vi "CCDAcqSingleSpectrum.vi"(0 "device selection":enum16{"monochromator", "CCD", "SCD"}(ring)=enum."CCD", 1 "ROI":T1, 5 "set-up a connection":bool=TRUE, 9 "tear down connection":bool=TRUE, 11 "error in":errorcluster, 12 "activate logger?":bool, 13 "Handler Name":string="example logger handler") -> (3 "log-file path":path, 6 "ROI cluster":T1, 15 "error out":errorcluster)   [LabVIEW 2023]
uses:
  Classes/CCD/CCDSpectralData.ctl
  Classes/CCD/XAxisConversionTypeEnum.ctl
  Classes/CCD/AcquisitionFormatEnum.ctl
  Classes/CCD/CCD.lvclass
  C:/Projects/Horiba/horiba-labview-sdk/Source/Classes/GenericDevice/GenericDevice.lvclass
  <vilib>/addons/_JKI Toolkits/Caraya/classes/Assert/Assert Not Error.vi
  <vilib>/addons/_JKI Toolkits/Caraya/classes/Test/Test.lvclass
  <vilib>/addons/_JKI Toolkits/Caraya/classes/Assert/Assert.lvclass
panel:
  # "Connector Pane"
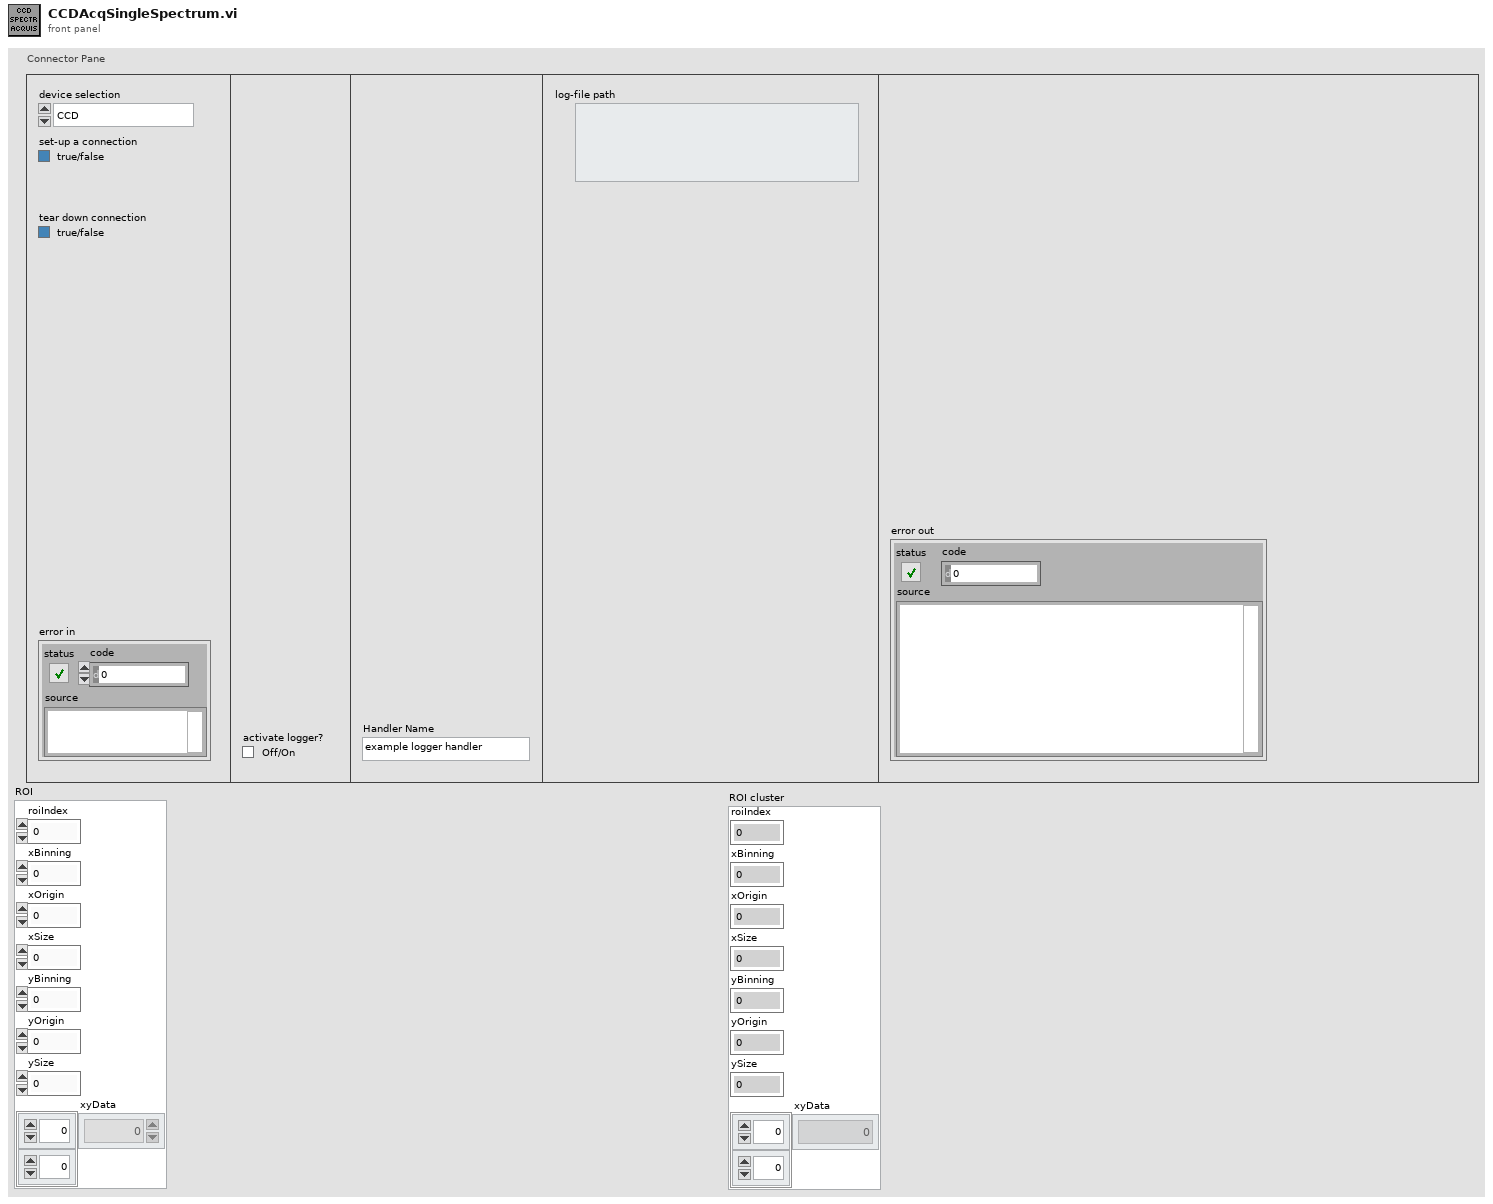
[diagram p1: front panel]
types:
  T1 = typedef "CCD.lvclass/CCDSpectralData.ctl" = cluster{"roiIndex":i32, "xBinning":i32, "xOrigin":i32, "xSize":i32, "yBinning":i32, "yOrigin":i32, "ySize":i32, "xyData":dbl[][]}
  T2 = typedef "CCD.lvclass/AcquisitionFormatEnum.ctl" = enum16{"Spectra", "Image", "Crop", "Fast Kinetics"}
  T3 = typedef "CCD.lvclass/XAxisConversionTypeEnum.ctl" = enum16{"None (default)", "CCD FIT parameters contained in the CCD firmware", "Mono Wavelength parameters contained in the icl_settings.ini file"}
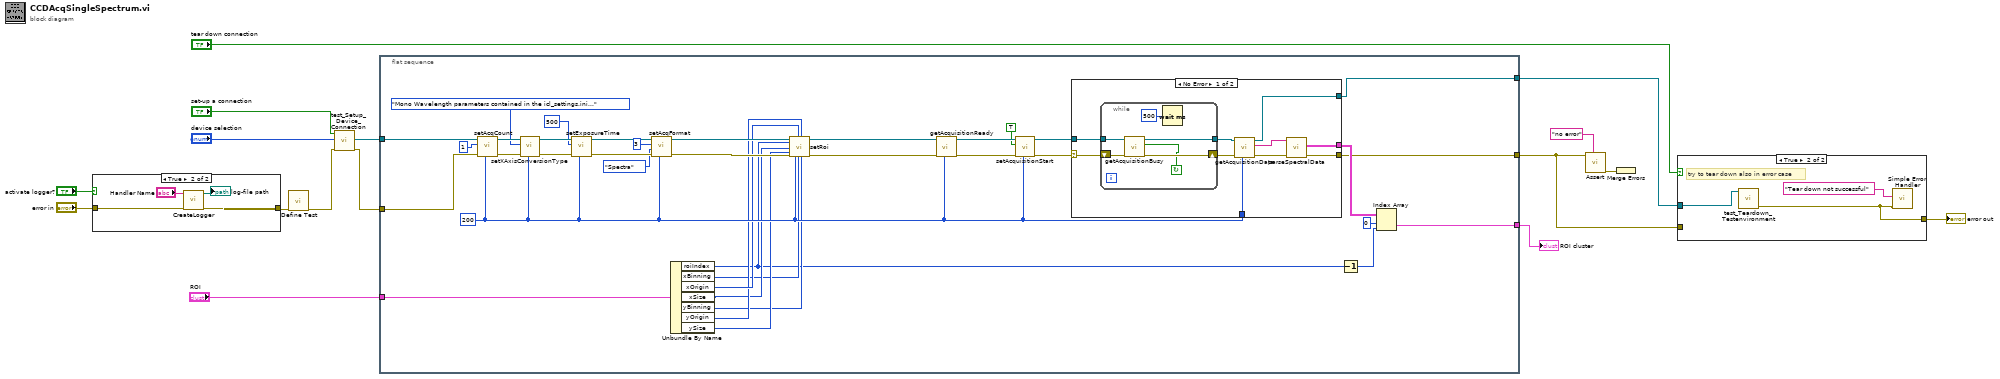
[diagram p0: block diagram]
diagram:
  n1 = case shown="True" "activate logger?" {
    tunnel: [w17 w20] -> w4
    tunnel: "error in" -> [w17 w21]
    frame False {
    }
    frame True {
      n2 = call "CreateLogger.vi"("error in (no error)"=w21, "Handler Name"="Handler Name") -> ("error out"=w20:errorcluster, "log-file path"=→"log-file path":path)  [unwired: 8 in]
    }
  }
  n3 = call <vilib>:"Define Test.vi"("error in (no error)"=w4) -> ("error out"=w9:errorcluster)  [unwired: 9 in, 1 out]
  n4 = call "test_Setup_Device_Connection.vi"("error in (no error)"=w9, "device selection"="device selection", "set-up a connection"="set-up a connection") -> ("error out"=w10:errorcluster, "CCD.lvclass"=w11:refnum<class "CCD.lvclass">)  [unwired: 5 in, 2 out]
  n5 = flat-sequence {
    tunnel: w10 -> [w57]
    tunnel: w11 -> [w58]
    tunnel: [w36] -> w13
    tunnel: [w46] -> w12
    tunnel: [w35] -> w3
    tunnel: "ROI" -> [w32]
    frame #0 {
      w33 = 200 ("Delay between send and receive [ms]")
      n6 = call "setAcqCount.vi"("Delay between send and receive [ms]"=w33, "error in (no error)"=w57, "count"=1, "CCD in"=w58) -> ("error out"=w54:errorcluster, "CCD out"=w55:refnum<class "CCD.lvclass">)  [unwired: 4 in, 2 out]
      n7 = call "setXAxisConversionType.vi"("Delay between send and receive [ms]"=w33, "error in (no error)"=w54, "Enum"=XAxisConversionTypeEnum."Mono Wavelength parameters contained in the icl_settings.ini file", "CCD in"=w55) -> ("error out"=w52:errorcluster, "CCD out"=w51:refnum<class "CCD.lvclass">)  [unwired: 4 in, 2 out]
      n8 = call "setExposureTime.vi"("Delay between send and receive [ms]"=w33, "error in (no error)"=w52, "exposure time [ms] or [us]"=500 ("exposure time [ms]"), "CCD in"=w51) -> ("error out"=w48:errorcluster, "CCD out"=w49:refnum<class "CCD.lvclass">)  [unwired: 4 in, 2 out]
      n9 = call "setAcqFormat.vi"("Delay between send and receive [ms]"=w33, "error in (no error)"=w48, "acquisition format"=AcquisitionFormatEnum."Spectra", "number of ROIs"=3, "CCD in"=w49) -> ("error out"=w44:errorcluster, "CCD out"=w45:refnum<class "CCD.lvclass">)  [unwired: 3 in, 2 out]
      n10 = Unbundle By Name(w32) -> ("roiIndex"=w23:i32, "xBinning"=w27:i32, "xOrigin"=w31:i32, "xSize"=w29:i32, "yBinning"=w26:i32, "yOrigin"=w30:i32, "ySize"=w28:i32)
      n11 = call "setRoi.vi"("CCD in"=w45, "ROI-index"=w23, "xSize"=w29, "ySize"=w28, "error in (no error)"=w44, "Delay between send and receive [ms]"=w33, "xOrigin"=w31, "xBin"=w27, "yOrigin"=w30, "yBin"=w26) -> ("CCD out"=w24:refnum<class "CCD.lvclass">, "error out"=w25:errorcluster)  [unwired: 6 in, 2 out]
      n12 = call "getAcquisitionReady.vi"("Delay between send and receive [ms]"=w33, "error in (no error)"=w25, "CCD in"=w24) -> ("error out"=w43:errorcluster, "CCD out"=w40:refnum<class "CCD.lvclass">)  [unwired: 6 in, 1 out]
      n13 = call "setAcquisitionStart.vi"("Delay between send and receive [ms]"=w33, "error in (no error)"=w43, "openShutter"=TRUE, "CCD in"=w40) -> ("error out"=w41:errorcluster, "CCD out"=w42:refnum<class "CCD.lvclass">)  [unwired: 4 in, 2 out]
      n14 = case shown="No Error" w41 {
        selector: w41 -> [w65 w75]
        tunnel: w42 -> [w68 w76]
        tunnel: [w64 w76] -> w46
        tunnel: [w62 w75] -> w36
        tunnel: [w60 _] -> w38
        tunnel: w33 -> [w59 _]
        frame No Error {
          n15 = while {
            tunnel: w68 -> [w74]
            tunnel: [w73] -> w67
            shift-right: [w71] -> w66
            shift-left: w65 -> [w70]
            stop <- w69 continue-if-true
            n16 = call "getAcquisitionBusy.vi"("error in (no error)"=w70, "CCD in"=w74) -> ("error out"=w71:errorcluster, "isBusy"=w69:bool, "CCD out"=w73:refnum<class "CCD.lvclass">)  [unwired: 7 in]
            n17 = Wait (ms)(milliseconds to wait=u32 500) -> ()  [unwired: 1 out]
          }
          n18 = call "getAcquisitionData.vi"("Delay between send and receive [ms]"=w59, "error in (no error)"=w66, "CCD in"=w67) -> ("error out"=w63:errorcluster, "results-JSON string"=w61:string, "CCD out"=w64:refnum<class "CCD.lvclass">)  [unwired: 6 in]
          n19 = call "parseSpectralData.vi"("error in (no error)"=w63, "results-JSON string"=w61) -> ("error out"=w62:errorcluster, "meta data"=w60:T1[][])  [unwired: 7 in, 1 out]
        }
        frame Error {
        }
      }
      n20 = Decrement(x=w23) -> (x-1=w22:i32)
      n21 = Index Array(array=w38, index (row)=0, index (col)=w22) -> (element=w35:T1)
    }
  }
  n22 = call-poly <vilib>:"Assert.vi"("Label"="no error" ("Label (VI Title)"), "Not Error?"=w13) -> ("error out"=w14:errorcluster)  [unwired: 8 in, 1 out]
  n23 = Merge Errors(w14) -> ()  [unwired: 1 out]
  n24 = case shown="True" "tear down connection" {
    tunnel: w12 -> [_ w79]
    tunnel: [w77 w78] -> w2
    tunnel: w13 -> [w77 _]
    frame False {
    }
    frame True {
      # "try to tear down also in error case"
      n25 = call "test_Teardown_Testenvironment.vi"("GenericDevice.lvclass"=w79) -> ("error out"=w78:errorcluster)  [unwired: 9 in, 1 out]
      n26 = call <vilib>:"Simple Error Handler.vi"("error source (\" \")"="Tear down not successful" ("error source (\" \")"), "error in (no error)"=w78) -> ()  [unwired: 3 in, 5 out]
    }
  }
  "error out" <- w2
  "ROI cluster" <- w3
